vi "TrainACC.vi"(6 "Min Index range":i32=2, 8 "Max Index range":i32=40, 9 "Contact":T4={"ID"=0, "UUID"="", "Name"="", "Iteration"=0, "Posit Array"=[], "Controls"={"throttle"=0.0, "brake"=0.0, "horn"=0.0, "wait"=0.5}, "DestArray"=[], "SetSpeed"=0.0, "Speed"=0.0, "PathData"={"Path Found?"=FALSE, "Same Line +Dir?"=FALSE, "Path"=[], "Distance to Dest"=0.0}}, 10 "Contacts":T4[](array[typedef]), 11 "All Lines":T1) -> (2 "Multiplier":dbl)   [LabVIEW 2014]
uses:
  Libraries/Contact Data/Contact.ctl
  Libraries/Contact Data/Position.ctl
  Libraries/Contact Data/Controls.ctl
  Libraries/Contact Data/DestinationCluster.ctl
  Libraries/Contact Data/DesinationControls.ctl
  Libraries/Contact Data/PathData.ctl
  PathFinder/Controls/ShortestPath.ctl
  Libraries/Map Data Folder/All-Lines.ctl
  Libraries/Map Data Folder/LineCluster.ctl
  Libraries/Map Data Folder/LineConnection.ctl
  Libraries/Map Data Folder/Map Data.lvlib
  Libraries/Contact Data/Contact Data.lvlib
panel:
  out "Name target":string
  out "Name":string
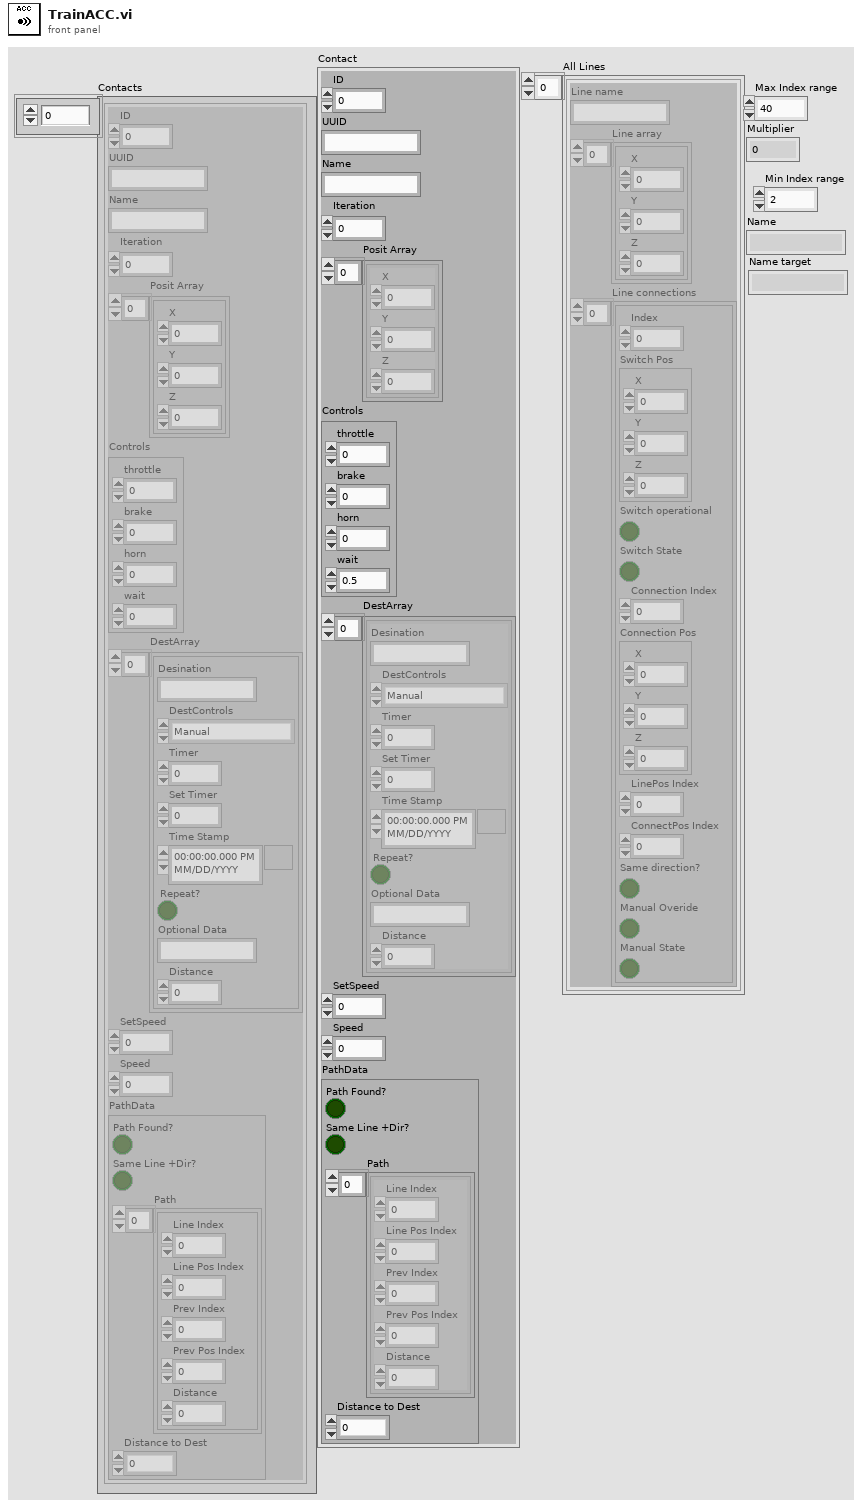
[diagram p1: front panel]
types:
  T1 = typedef "Map Data.lvlib/All-Lines.ctl" = T2[]
  T2 = typedef "Map Data.lvlib/LineCluster.ctl" = cluster{"Line name":string, "Line array":cluster{"X":dbl, "Y":dbl, "Z":dbl}[], "Line connections":T3[]}
  T3 = typedef "Map Data.lvlib/LineConnection.ctl" = cluster{"Index":i32, "Switch Pos":cluster{"X":dbl, "Y":dbl, "Z":dbl}, "Switch operational":bool, "Switch State":bool, "Connection Index":i32, "Connection Pos":cluster{"X":dbl, "Y":dbl, "Z":dbl}, "LinePos Index":i32, "ConnectPos Index":i32, "Same direction?":bool, "Manual Overide":bool, "Manual State":bool}
  T4 = typedef "Contact Data.lvlib/Contact.ctl" = cluster{"ID":u32, "UUID":string, "Name":string, "Iteration":i32, "Posit Array":T5[], "Controls":T6, "DestArray":T7[], "SetSpeed":dbl, "Speed":dbl, "PathData":T9}
  T5 = typedef "Contact Data.lvlib/Position.ctl" = cluster{"X":dbl, "Y":dbl, "Z":dbl}
  T6 = typedef "Contact Data.lvlib/Controls.ctl" = cluster{"throttle":dbl, "brake":dbl, "horn":dbl, "wait":dbl}
  T7 = typedef "Contact Data.lvlib/DestinationCluster.ctl" = cluster{"Desination":string, "DestControls":T8, "Timer":u32, "Set Timer":u32, "Time Stamp":timestamp, "Repeat?":bool, "Optional Data":string, "Distance":dbl}
  T8 = typedef "Contact Data.lvlib/DesinationControls.ctl" = enum16{"Tracker", "Manual", "Stop", "Station DateTime", "Station Timer", "Maintain"}
  T9 = typedef "Contact Data.lvlib/PathData.ctl" = cluster{"Path Found?":bool, "Same Line +Dir?":bool, "Path":T10[], "Distance to Dest":dbl}
  T10 = typedef "ShortestPath.ctl" = cluster{"Line Index":i32, "Line Pos Index ":i32, "Prev Index ":i32, "Prev Pos Index":i32, "Distance":dbl}
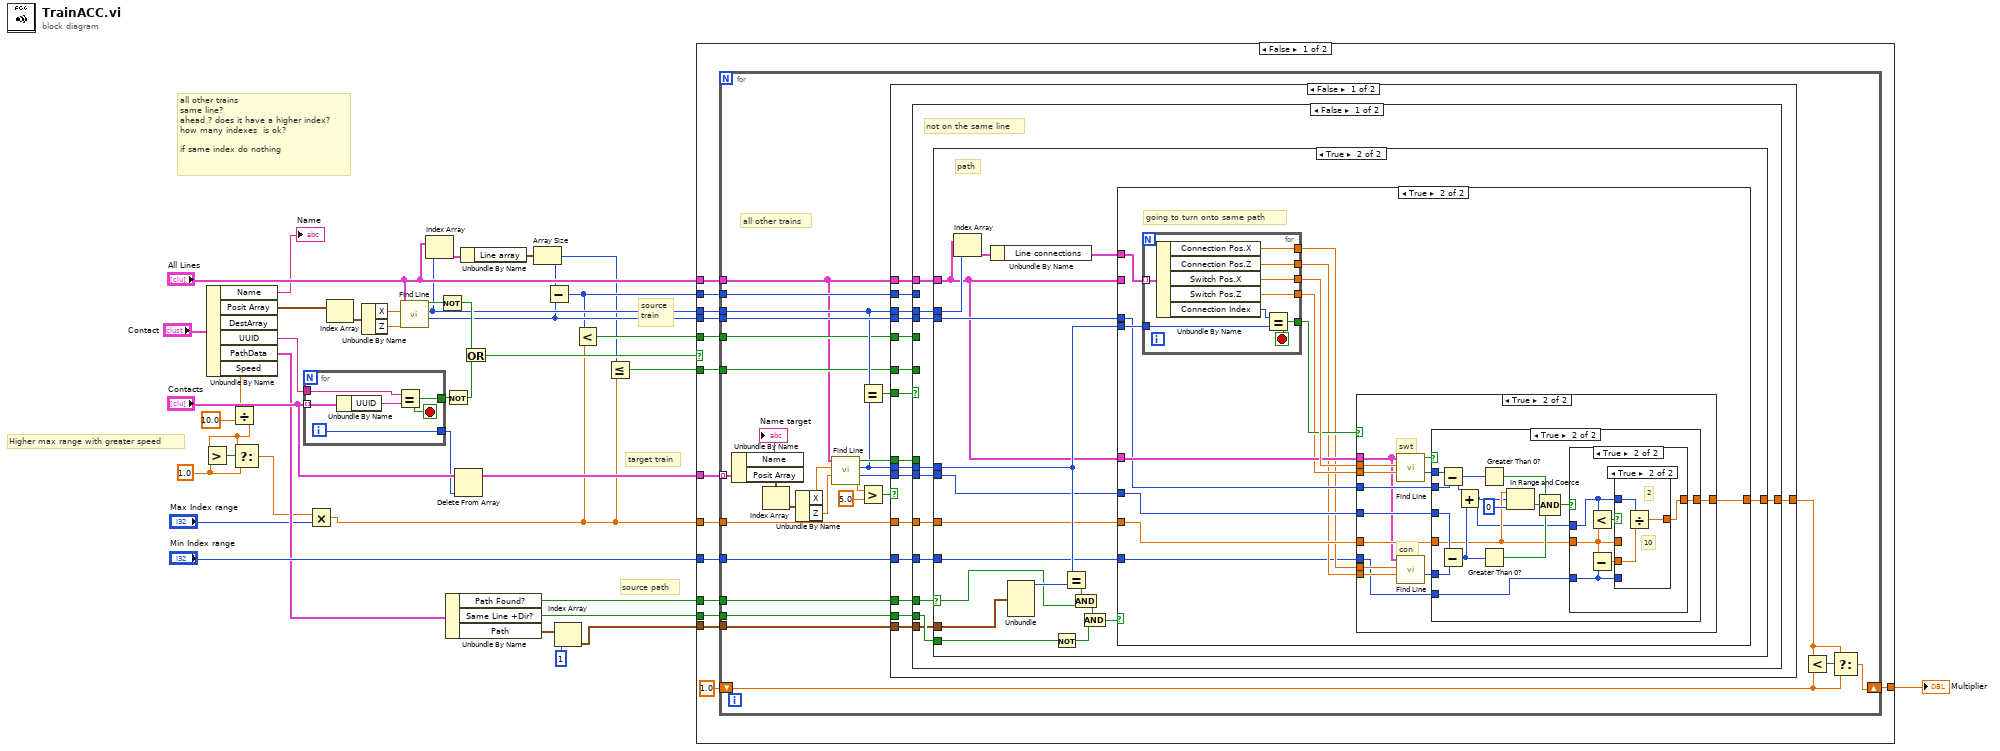
[diagram p0: block diagram]
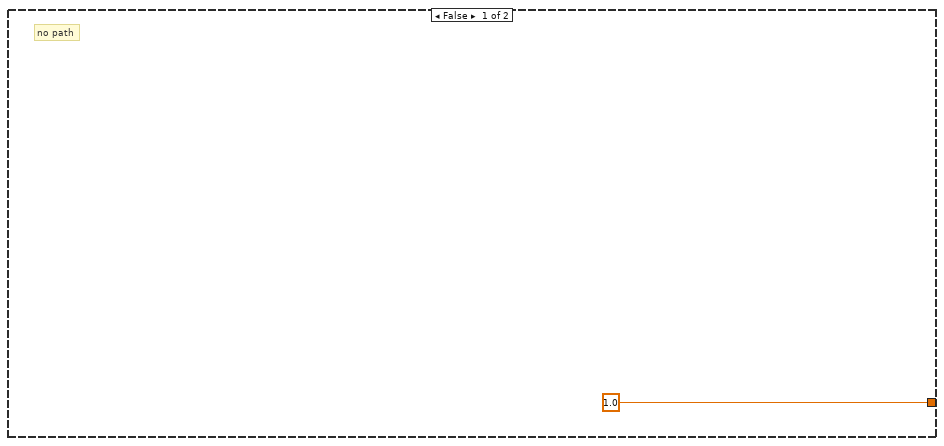
[diagram p2: hidden frame]
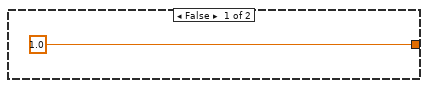
[diagram p3: hidden frame]
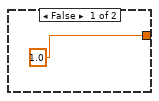
[diagram p4: hidden frame]
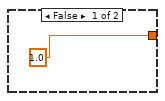
[diagram p5: hidden frame]
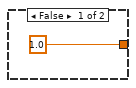
[diagram p6: hidden frame]
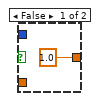
[diagram p7: hidden frame]
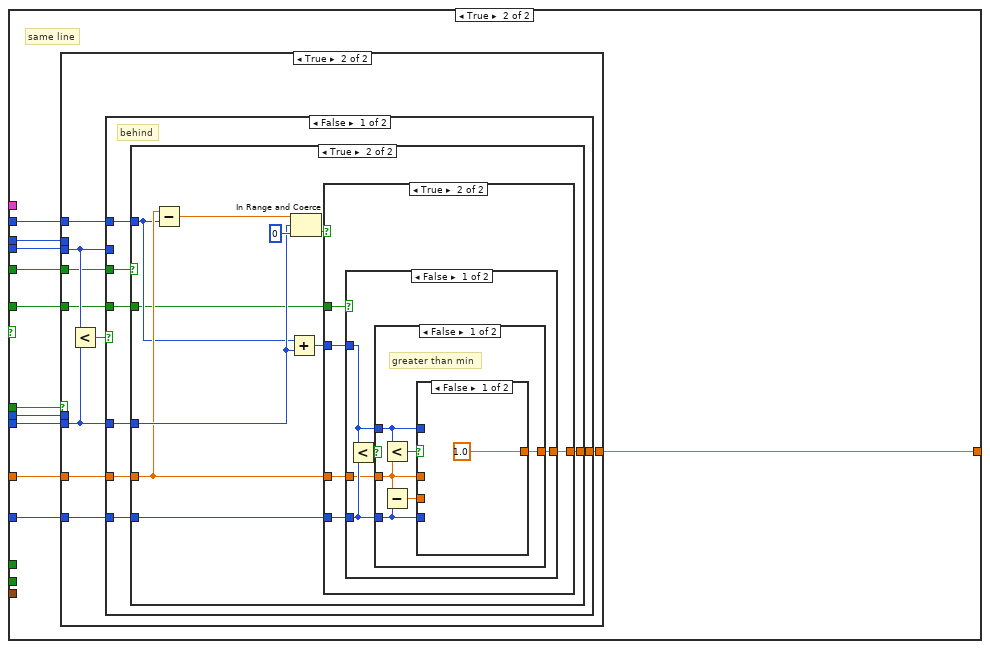
[diagram p8: hidden frame]
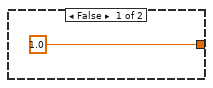
[diagram p9: hidden frame]
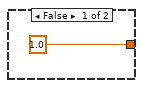
[diagram p10: hidden frame]
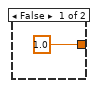
[diagram p11: hidden frame]
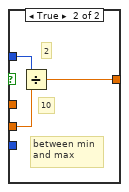
[diagram p12: hidden frame]
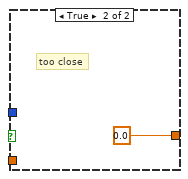
[diagram p13: hidden frame]
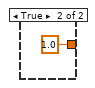
[diagram p14: hidden frame]
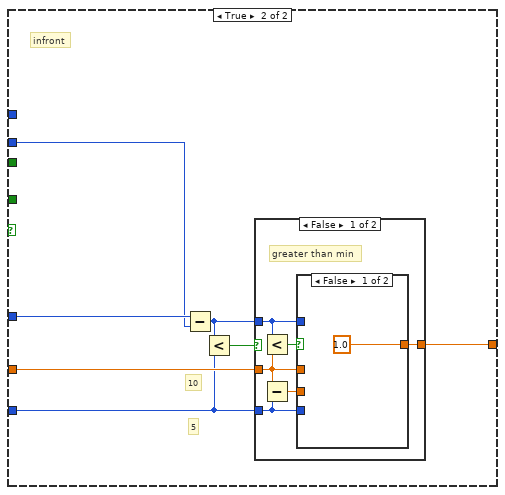
[diagram p15: hidden frame]
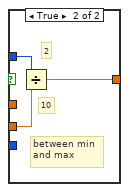
[diagram p16: hidden frame]
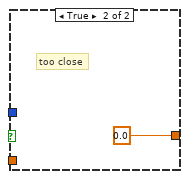
[diagram p17: hidden frame]
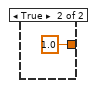
[diagram p18: hidden frame]
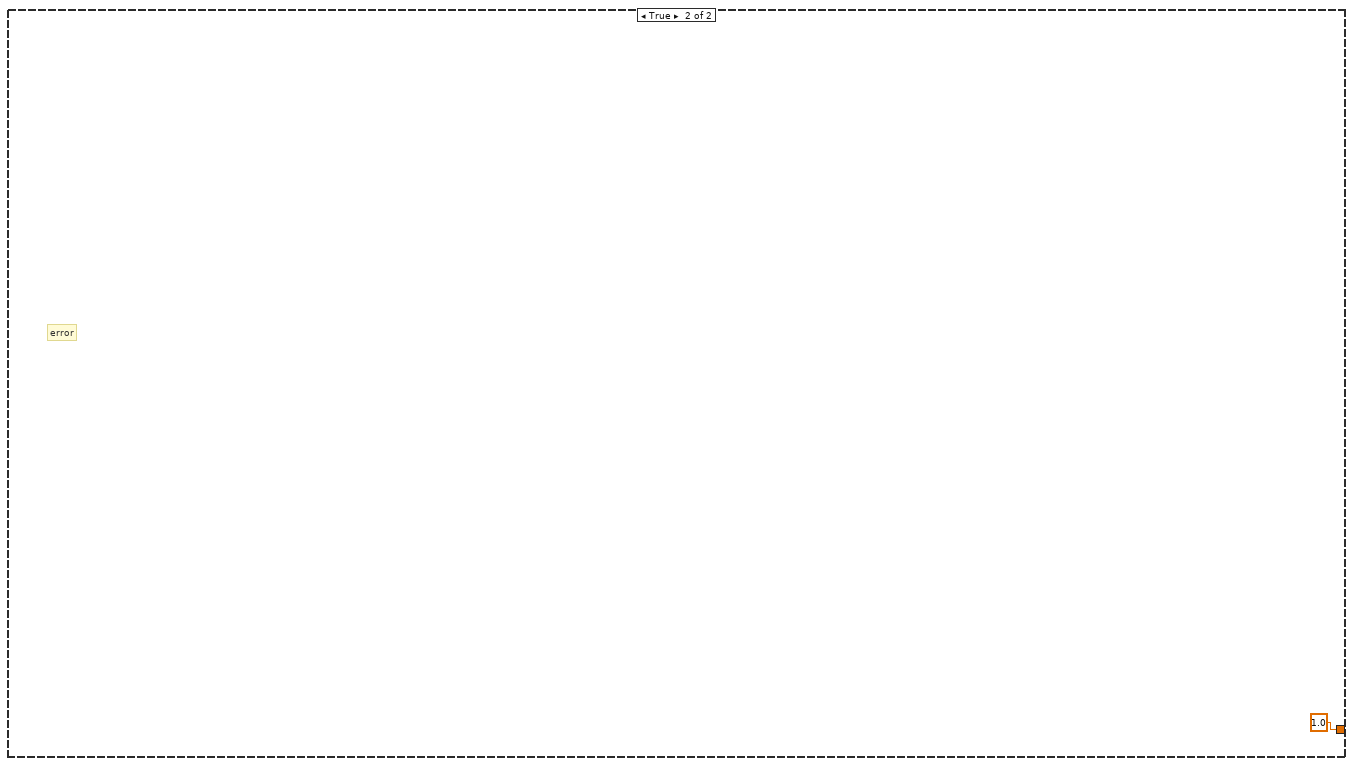
[diagram p19: hidden frame]
diagram:
  w5 = 1.0 ("y")
  # "source path"
  # "source\ntrain"
  # "target train"
  # "Higher max range with greater speed"
  # "all other trains\nsame line?\nahead ? does it have a higher index?\nhow many indexes  is ok?\n\nif same index do nothing"
  n1 = Unbundle By Name("Contact") -> ("Name"=→"Name":string, "Posit Array"=w16:T5[], "UUID"=w21:string, "PathData"=w15:T9, "Speed"=w9:dbl)  [unwired: 1 out]
  n2 = Divide(x=w9, y=10.0) -> (x/y=w4:dbl)
  n3 = Greater?(x=w4, y=w5) -> (0:w6:bool)
  n4 = Select(t=w4, s=w6, f=w5) -> (s? t:f=w3:dbl)
  n5 = for {
    tunnel: "Contacts" -> [w45] mode=indexing
    tunnel: [w44] -> w36
    tunnel: [w43] -> w38
    tunnel: w21 -> [w41]
    i -> [w43]
    stop <- w44 stop-if-true
    n6 = Unbundle By Name(w45) -> ("UUID"=w42:string)
    n7 = Equal?(x=w41, y=w42) -> (x = y?=w44:bool)
  }
  n8 = Multiply(x=w3, y="Max Index range") -> (x*y=w1:dbl)
  n9 = Index Array(array=w16) -> (element=w19:T5)  [unwired: 1 in]
  n10 = Unbundle By Name(w19) -> ("X"=w18:dbl, "Z"=w17:dbl)
  n11 = call "Find Line.vi"("Z"=w17, "X"=w18, "All Lines"="All Lines") -> ("Index on Line"=w25:i32, "Nearest Line"=w28:i32, "Line found?"=w35:bool)  [unwired: 5 in, 1 out]
  n12 = Index Array(array="All Lines", index=w28) -> (element=w27:T2)
  n13 = Not(x=w35) -> (.not. x?=w33:bool)
  n14 = Not(x=w36) -> (.not. x?=w34:bool)
  n15 = Unbundle By Name(w15) -> ("Path Found?"=w14:bool, "Same Line +Dir?"=w13:bool, "Path"=w12:T10[])
  n16 = Delete From Array(array="Contacts", index=w38) -> (array with subset deleted=w37:T4[])  [unwired: 1 in, 1 out]
  n17 = Unbundle By Name(w27) -> ("Line array"=w26:cluster{"X":dbl, "Y":dbl, "Z":dbl}[])
  n18 = Or(x=w33, y=w34) -> (x .or. y?=w32:bool)
  n19 = Array Size(array=w26) -> (size(s)=w20:i32)
  n20 = Subtract(x=w20, y=w25) -> (x-y=w23:i32)
  n21 = Index Array(array=w12, index=1) -> (element=w10:T10)
  n22 = Less?(x=w23, y=w1) -> (x < y?=w24:bool)
  n23 = Less Or Equal?(x=w20, y=w1) -> (x <= y?=w22:bool)
  n24 = case shown="False" w32 {
    tunnel: w37 -> [w59 _]
    tunnel: w25 -> [w58 _]
    tunnel: w28 -> [w57 _]
    tunnel: "All Lines" -> [w56 _]
    tunnel: w1 -> [w55 _]
    tunnel: [w53 1.0] -> w31
    tunnel: "Min Index range" -> [w52 _]
    tunnel: w24 -> [w51 _]
    tunnel: w23 -> [w50 _]
    tunnel: w22 -> [w49 _]
    tunnel: w14 -> [w48 _]
    tunnel: w13 -> [w47 _]
    tunnel: w10 -> [w46 _]
    frame False {
      n25 = for {
        tunnel: w59 -> [w87] mode=indexing
        tunnel: w58 -> [w84]
        tunnel: w57 -> [w77]
        tunnel: w56 -> [w70]
        tunnel: w55 -> [w83]
        shift-right: [w79] -> w53
        shift-left: 1.0 -> [w80]
        tunnel: w52 -> [w75]
        tunnel: w51 -> [w74]
        tunnel: w50 -> [w73]
        tunnel: w49 -> [w72]
        tunnel: w48 -> [w71]
        tunnel: w47 -> [w65]
        tunnel: w46 -> [w64]
        # "all other trains"
        n26 = Unbundle By Name(w87) -> ("Name"=→"Name target":string, "Posit Array"=w68:T5[])
        n27 = Index Array(array=w68) -> (element=w69:T5)  [unwired: 1 in]
        n28 = Unbundle By Name(w69) -> ("X"=w67:dbl, "Z"=w66:dbl)
        n29 = call "Find Line.vi"("Z"=w66, "X"=w67, "All Lines"=w70) -> ("Distance to nearest"=w62:dbl, "Index on Line"=w85:i32, "Nearest Line"=w78:i32, "Line found?"=w86:bool)  [unwired: 5 in]
        n30 = Equal?(x=w77, y=w78) -> (x = y?=w76:bool)
        n31 = Greater?(x=w62, y=5.0) -> (0:w60:bool)
        n32 = case shown="False" w60 {
          tunnel: w86 -> [w103 _]
          tunnel: w85 -> [w102 _]
          tunnel: w84 -> [w101 _]
          tunnel: w83 -> [w100 _]
          tunnel: [w99 1.0] -> w81
          tunnel: w78 -> [w98 _]
          tunnel: w77 -> [w97 _]
          tunnel: w76 -> [w96 _]
          tunnel: w75 -> [w95 _]
          tunnel: w74 -> [w94 _]
          tunnel: w73 -> [w93 _]
          tunnel: w72 -> [w92 _]
          tunnel: w71 -> [w91 _]
          tunnel: w70 -> [w90 _]
          tunnel: w65 -> [w89 _]
          tunnel: w64 -> [w88 _]
          frame False {
            n33 = case shown="False" w96 {
              tunnel: w103 -> [_ w207]
              tunnel: w102 -> [w111 w206]
              tunnel: w101 -> [w112 w205]
              tunnel: w100 -> [w110 w204]
              tunnel: [w114 w203] -> w99
              tunnel: w98 -> [w113 w202]
              tunnel: w97 -> [w109 w201]
              tunnel: w95 -> [w106 w200]
              tunnel: w94 -> [_ w199]
              tunnel: w93 -> [_ w198]
              tunnel: w92 -> [_ w197]
              tunnel: w91 -> [w107 _]
              tunnel: w90 -> [w108 _]
              tunnel: w89 -> [w105 _]
              tunnel: w88 -> [w104 _]
              frame False {
                # "not on the same line"
                n34 = case shown="True" w107 {
                  selector: w107 -> [_ w118]
                  tunnel: [1.0 w132] -> w114
                  tunnel: w113 -> [_ w131]
                  tunnel: w112 -> [_ w130]
                  tunnel: w111 -> [_ w129]
                  tunnel: w110 -> [_ w128]
                  tunnel: w109 -> [_ w127]
                  tunnel: w108 -> [_ w126]
                  tunnel: w106 -> [_ w120]
                  tunnel: w105 -> [_ w117]
                  tunnel: w104 -> [_ w116]
                  frame False {
                    # "no path"
                  }
                  frame True {
                    # "path"
                    n35 = Index Array(array=w126, index=w127) -> (element=w125:T2)
                    n36 = Unbundle By Name(w125) -> ("Line connections"=w124:T3[])
                    n37 = Unbundle(w116) -> ("Line Index"=w119:i32)  [unwired: 4 out]
                    n38 = Not(x=w117) -> (.not. x?=w121:bool)
                    n39 = Equal?(x=w131, y=w119) -> (x = y?=w133:bool)
                    n40 = And(x=w133, y=w118) -> (x .and. y?=w123:bool)
                    n41 = And(x=w123, y=w121) -> (x .and. y?=w122:bool)
                    n42 = case shown="True" w122 {
                      tunnel: [1.0 w140] -> w132
                      tunnel: w126 -> [_ _]
                      tunnel: w131 -> [_ w147]
                      tunnel: w126 -> [_ w144]
                      tunnel: w130 -> [_ w143]
                      tunnel: w129 -> [_ w142]
                      tunnel: w128 -> [_ w141]
                      tunnel: w124 -> [_ w139]
                      tunnel: w120 -> [_ w135]
                      frame False {
                      }
                      frame True {
                        # "going to turn onto same path"
                        n43 = for {
                          tunnel: w139 -> [w196] mode=indexing
                          tunnel: w147 -> [w195]
                          tunnel: [w194] -> w138
                          tunnel: [w193] -> w146
                          tunnel: [w192] -> w145
                          tunnel: [w190] -> w136
                          tunnel: [w189] -> w137
                          stop <- w192 stop-if-true
                          n44 = Unbundle By Name(w196) -> ("Connection Pos.X"=w189:dbl, "Connection Pos.Z"=w190:dbl, "Switch Pos.X"=w193:dbl, "Switch Pos.Z"=w194:dbl, "Connection Index"=w191:i32)
                          n45 = Equal?(x=w191, y=w195) -> (x = y?=w192:bool)
                        }
                        n46 = case shown="True" w145 {
                          tunnel: w146 -> [_ w155]
                          tunnel: w144 -> [_ w153]
                          tunnel: w143 -> [_ w159]
                          tunnel: w142 -> [_ w158]
                          tunnel: w141 -> [_ w157]
                          tunnel: [1.0 w156] -> w140
                          tunnel: w138 -> [_ w154]
                          tunnel: w137 -> [_ w152]
                          tunnel: w136 -> [_ w151]
                          tunnel: w135 -> [_ w149]
                          frame False {
                          }
                          frame True {
                            # "con"
                            # "swt"
                            n47 = call "Find Line.vi"("Z"=w154, "X"=w155, "All Lines"=w153) -> ("Index on Line"=w160:i32, "Line found?"=w161:bool)  [unwired: 5 in, 2 out]
                            n48 = call "Find Line.vi"("Z"=w151, "X"=w152, "All Lines"=w153) -> ("Index on Line"=w150:i32)  [unwired: 5 in, 3 out]
                            n49 = case shown="True" w161 {
                              tunnel: w160 -> [_ w172]
                              tunnel: w159 -> [_ w173]
                              tunnel: w158 -> [_ w174]
                              tunnel: w157 -> [_ w165]
                              tunnel: [1.0 w176] -> w156
                              tunnel: w150 -> [_ w175]
                              tunnel: w149 -> [_ w164]
                              frame False {
                              }
                              frame True {
                                n50 = Subtract(x=w172, y=w173) -> (x-y=w171:i32)
                                n51 = Subtract(x=w174, y=w175) -> (x-y=w170:i32)
                                n52 = Add(x=w171, y=w170) -> (x+y=w163:i32)
                                n53 = Greater Than 0?(x=w171) -> (x > 0?=w167:bool)
                                n54 = Greater Than 0?(x=w170) -> (x > 0?=w166:bool)
                                n55 = In Range and Coerce(upper limit=w165, x=w163, lower limit=0) -> (In Range?=w169:bool)  [unwired: 1 out]
                                n56 = Compound Arithmetic op=AND(w167, w169, w166) -> (w168:bool)
                                n57 = case shown="True" w168 {
                                tunnel: [1.0 w179] -> w176
                                tunnel: w165 -> [_ w182]
                                tunnel: w164 -> [_ w181]
                                tunnel: w163 -> [_ w180]
                                frame False {
                                }
                                frame True {
                                n58 = Less?(x=w180, y=w182) -> (x < y?=w184:bool)
                                n59 = Subtract(x=w182, y=w181) -> (x-y=w183:dbl)
                                n60 = case shown="True" w184 {
                                tunnel: w180 -> [_ w188]
                                tunnel: w182 -> [_ _]
                                tunnel: [1.0 w187] -> w179
                                tunnel: w181 -> [_ _]
                                tunnel: w183 -> [_ w186]
                                frame False {
                                }
                                frame True {
                                # "2"
                                # "10"
                                n61 = Divide(x=w188, y=w186) -> (x/y=w187:dbl)
                                }
                                }
                                }
                                }
                              }
                            }
                          }
                        }
                      }
                    }
                  }
                }
              }
              frame True {
                # "same line"
                n62 = case shown="True" w207 {
                  tunnel: w202 -> [_ _]
                  tunnel: w206 -> [_ w217]
                  tunnel: w201 -> [_ _]
                  tunnel: w205 -> [_ w216]
                  tunnel: w204 -> [_ w215]
                  tunnel: [1.0 w214] -> w203
                  tunnel: w200 -> [_ w213]
                  tunnel: w199 -> [_ w212]
                  tunnel: w198 -> [_ w211]
                  tunnel: w197 -> [_ w209]
                  frame False {
                  }
                  frame True {
                    n63 = Less?(x=w216, y=w217) -> (x < y?=w210:bool)
                    n64 = case shown="False" w210 {
                      tunnel: w217 -> [w222 w265]
                      tunnel: w216 -> [_ w264]
                      tunnel: w215 -> [w220 w262]
                      tunnel: [w224 w263] -> w214
                      tunnel: w213 -> [w219 w260]
                      tunnel: w212 -> [w223 _]
                      tunnel: w211 -> [w221 _]
                      tunnel: w209 -> [w218 _]
                      frame False {
                        # "behind"
                        n65 = case shown="True" w223 {
                          tunnel: [1.0 w229] -> w224
                          tunnel: w222 -> [_ w232]
                          tunnel: w221 -> [_ w227]
                          tunnel: w220 -> [_ w228]
                          tunnel: w219 -> [_ w230]
                          tunnel: w218 -> [_ w226]
                          frame False {
                          }
                          frame True {
                            n66 = Subtract(x=w228, y=w227) -> (x-y=w235:dbl)
                            n67 = Add(x=w227, y=w232) -> (x+y=w231:i32)
                            n68 = In Range and Coerce(upper limit=w235, x=w232, lower limit=0) -> (In Range?=w233:bool)  [unwired: 1 out]
                            n69 = case shown="True" w233 {
                              tunnel: w231 -> [_ w241]
                              tunnel: w230 -> [_ w240]
                              tunnel: w228 -> [_ w239]
                              tunnel: [1.0 w238] -> w229
                              tunnel: w226 -> [_ w237]
                              frame False {
                              }
                              frame True {
                                n70 = case shown="False" w237 {
                                tunnel: w241 -> [w245 _]
                                tunnel: w240 -> [w244 _]
                                tunnel: w239 -> [w243 _]
                                tunnel: [w242 1.0] -> w238
                                frame False {
                                n71 = Less?(x=w245, y=w244) -> (x < y?=w246:bool)
                                n72 = case shown="False" w246 {
                                tunnel: [w251 0.0] -> w242
                                tunnel: w243 -> [w250 _]
                                tunnel: w245 -> [w248 _]
                                tunnel: w244 -> [w247 _]
                                frame False {
                                # "greater than min"
                                n73 = Less?(x=w248, y=w250) -> (x < y?=w252:bool)
                                n74 = Subtract(x=w250, y=w247) -> (x-y=w249:dbl)
                                n75 = case shown="False" w252 {
                                tunnel: w248 -> [_ w256]
                                tunnel: w250 -> [_ _]
                                tunnel: [1.0 w255] -> w251
                                tunnel: w247 -> [_ _]
                                tunnel: w249 -> [_ w254]
                                frame False {
                                }
                                frame True {
                                # "between min\nand max"
                                # "2"
                                # "10"
                                n76 = Divide(x=w256, y=w254) -> (x/y=w255:dbl)
                                }
                                }
                                }
                                frame True {
                                # "too close"
                                }
                                }
                                }
                                frame True {
                                }
                                }
                              }
                            }
                          }
                        }
                      }
                      frame True {
                        # "infront"
                        # "5"
                        # "10"
                        n77 = Subtract(x=w265, y=w264) -> (x-y=w261:i32)
                        n78 = Less?(x=w261, y=w260) -> (x < y?=w259:bool)
                        n79 = case shown="False" w259 {
                          tunnel: [w270 0.0] -> w263
                          tunnel: w262 -> [w269 _]
                          tunnel: w261 -> [w267 _]
                          tunnel: w260 -> [w266 _]
                          frame False {
                            # "greater than min"
                            n80 = Less?(x=w267, y=w269) -> (x < y?=w271:bool)
                            n81 = Subtract(x=w269, y=w266) -> (x-y=w268:dbl)
                            n82 = case shown="False" w271 {
                              tunnel: w267 -> [_ w275]
                              tunnel: w269 -> [_ _]
                              tunnel: [1.0 w274] -> w270
                              tunnel: w266 -> [_ _]
                              tunnel: w268 -> [_ w273]
                              frame False {
                              }
                              frame True {
                                # "between min\nand max"
                                # "2"
                                # "10"
                                n83 = Divide(x=w275, y=w273) -> (x/y=w274:dbl)
                              }
                            }
                          }
                          frame True {
                            # "too close"
                          }
                        }
                      }
                    }
                  }
                }
              }
            }
          }
          frame True {
          }
        }
        n84 = Less?(x=w81, y=w80) -> (x < y?=w82:bool)
        n85 = Select(t=w81, s=w82, f=w80) -> (s? t:f=w79:dbl)
      }
    }
    frame True {
      # "error"
    }
  }
  "Multiplier" <- w31
